vi "SystemToggleMagBrakeControl (1).vi"(11 "MagBrakeOn?":bool) -> (3 "MagBrakeToggle Complete":bool)   [LabVIEW 2017]
doc: "Enables or disables Magnetic Braking in optimal order to prevent unneccessary air loss. Also ensures that, when present, pressure will remain above desired level."
uses:
  Sensors/DataStreamIndex.ctl
  DataTargetsGLOBAL.vi
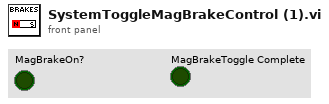
[diagram p1: front panel]
types:
  T1 = typedef "DataStreamIndex.ctl" = enum16{"SuspensionPT (PSI)", "MagBrakePT (PSI)", "Baby HPPT (PSI)", "BigRight HPPT (PSI)", "BigLeft HPPT (PSI)", "HallEffect FrontLeft (V)", "HallEffect FrontRight (V)", "HallEffect BackRight (V)", "HallEffect BackLeft (V)", "LinearPot FrontRight (V)", "LinearPot FrontLeft (V)", "LinearPot BackRight (V)", "LinearPot BackLeft (V)", "Speed (m/s)", "Distance (m)", "Piezo (V)", "Battery Voltage (V)", "Battery Current", "Battery Temperature (C)", "cRIO Temperature (C)", "Right Big Tank Temperature (C)", "Left Big Tank Temperature (C)", "Baby Tank Temperature (C)", "Right Manifold Temperature (C)", "Left Manifold Temperature (C)", "IMU Acceleration (m/s2)", "IMU Pressure (Pa)", "IMU Temperature (C)"}
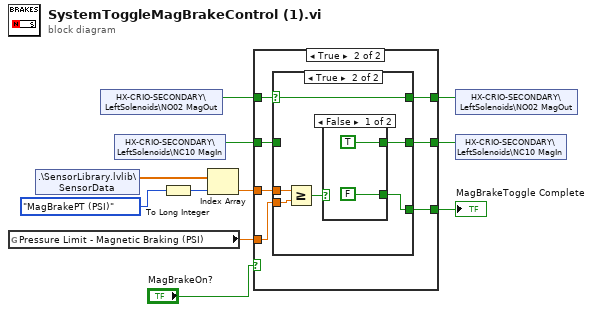
[diagram p0: block diagram]
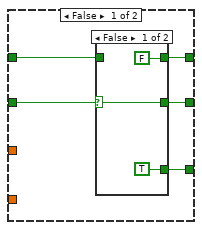
[diagram p2: hidden frame]
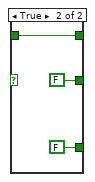
[diagram p3: hidden frame]
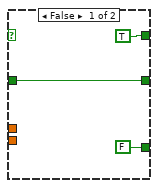
[diagram p4: hidden frame]
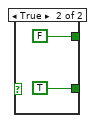
[diagram p5: hidden frame]
diagram:
  n1 = global read "DataTargetsGLOBAL.vi" "Pressure Limit - Magnetic Braking (PSI)"() -> (w5:dbl)
  n2 = shared-variable ".\\SensorLibrary.lvlib\\SensorData"() -> (w4:dbl[])  [unwired: 1 in, 1 out]
  n3 = shared-variable "HX-CRIO-SECONDARY\\LeftSolenoids\\NO02 MagOut"() -> (w9:bool)  [unwired: 1 in, 1 out]
  n4 = shared-variable "HX-CRIO-SECONDARY\\LeftSolenoids\\NC10 MagIn"() -> (w8:bool)  [unwired: 1 in, 1 out]
  n5 = To Long Integer(number=DataStreamIndex."MagBrakePT (PSI)" ("Data Stream Index")) -> (32bit integer=w2:i32)
  n6 = Index Array(array=w4, index=w2) -> (element=w3:dbl)
  n7 = case shown="True" "MagBrakeOn?" {
    tunnel: w9 -> [w13 w29]
    tunnel: [w14 w28] -> w6
    tunnel: [w15 w27] -> w7
    tunnel: w8 -> [w16 w26]
    tunnel: w5 -> [_ w25]
    tunnel: w3 -> [_ w24]
    tunnel: [w12 w23] -> w10
    frame False {
      n8 = case shown="False" w16 {
        selector: w16 -> [w18 _]
        tunnel: [w18 FALSE] -> w15
        tunnel: [FALSE ("MagBrake OUTPUT") w21] -> w14
        tunnel: w13 -> [_ w21]
        tunnel: [TRUE FALSE] -> w12
        frame False {
        }
        frame True {
        }
      }
    }
    frame True {
      n9 = case shown="True" w29 {
        selector: w29 -> [_ w38]
        tunnel: [TRUE w38] -> w28
        tunnel: [w31 w36] -> w27
        tunnel: w26 -> [w31 _]
        tunnel: w25 -> [_ w37]
        tunnel: w24 -> [_ w35]
        tunnel: [FALSE w34] -> w23
        frame False {
        }
        frame True {
          n10 = Greater Or Equal?(x=w35, y=w37) -> (x >= y?=w33:bool)
          n11 = case shown="False" w33 {
            tunnel: [TRUE FALSE] -> w36
            tunnel: [FALSE TRUE] -> w34
            frame False {
            }
            frame True {
            }
          }
        }
      }
    }
  }
  "MagBrakeToggle Complete" <- w10
  n12 = shared-variable "HX-CRIO-SECONDARY\\LeftSolenoids\\NO02 MagOut"(w6) -> ()  [unwired: 1 in, 1 out]
  n13 = shared-variable "HX-CRIO-SECONDARY\\LeftSolenoids\\NC10 MagIn"(w7) -> ()  [unwired: 1 in, 1 out]
